vi "fgt get sensor Channel Count.vi"(8 "error in (no error)":errorcluster) -> (0 "error out":errorcluster, 3 "nbSChan out":u32)   [LabVIEW 2016, in "fgt_SDK.lvlib"]
doc: "Get total number of initialized sensor channels.\nIt is the sum of all connected flow-units on Flowboard, FlowEZ and IPS sensors"
uses:
  fgt_SDK.lvlib
  dlls/fgt_SDK_32.dll
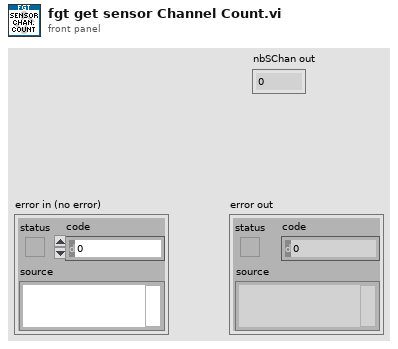
[diagram p1: front panel]
types:
  T1 = typedef "fgt_SDK.lvlib/fgt_STATUS_INFO.ctl" = cluster{"InstrType":T2, "instrSN":u16, "errorCode":u8, "infoCode":u8, "detail":string}
  T2 = typedef "fgt_SDK.lvlib/fgt_INSTRUMENT_TYPE.ctl" = enum32{"None", "MFCS", "MFCS_EZ", "FRP", "LineUP", "IPS"}
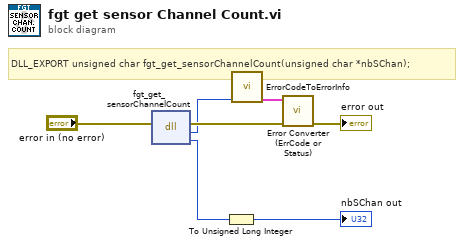
[diagram p0: block diagram]
diagram:
  # "DLL_EXPORT unsigned char fgt_get_sensorChannelCount(unsigned char *nbSChan);"
  n1 = dll-call lib="C:/projects/SDK/fgt-sdk-labview/dlls/fgt_SDK_*.*" fn="fgt_get_sensorChannelCount"(error in="error in (no error)") -> (error out=w6:errorcluster, "return type"=w4:u8, "nbSChan"=w2:u8)  [unwired: 3 in, 1 out]
  n2 = To Unsigned Long Integer(number=w2) -> (unsigned 32bit integer=→"nbSChan out":u32)
  n3 = call "ErrorCodeToErrorInfo.vi"("return type"=w4) -> ("StatusInfo"=w3:T1)  [unwired: 10 in]
  n4 = call "Error Converter (ErrCode or Status).vi"("error in (no error)"=w6, "StatusInfo"=w3) -> ("error out"=→"error out":errorcluster)  [unwired: 9 in]
